vi "testcases.vi"() -> ()   [LabVIEW 2025]
uses:
  <vilib>/LabVIEW Interface for Arduino/Type Defs/Pin Mode.ctl
  <vilib>/LabVIEW Interface for Arduino/LabVIEW Interface for Arduino.lvlib
panel:
  in  "stop":bool
  out "error out":errorcluster
  in  "Board":refnum<visa-resource-name>
  in  "Test cases":T1(ring)
  in  "Tab Control":T2(tab)
  in  "pin":u8
  in  "input val":u8
  out "Value":u8
  out "Outputs":bool[](array[boolean])
  in  "Set values":bool[](array[boolean])
  out "Voltage":dbl(knob) scale=0.0..5.0
  in  "Analog Input Pin (0)":u8
  out "Analog Port":dbl[](array[numeric])
  out "Waveform Chart":dbl(graph)
  in  "PWM 0 (0-255)":u8
  in  "PWM 1 (0-255)":u8
  in  "PWM 2 (0-255)":u8
  in  "PWM Pins":u8[](array[numeric])
  in  "Analog Input Pin":u8
  in  "pwm write single":u8
  in  "PWM Pin single":u8=3
  # "Arduino v4 tests"
  # "0x00 and 0x01 definitely work since every other case requires init and close to function"
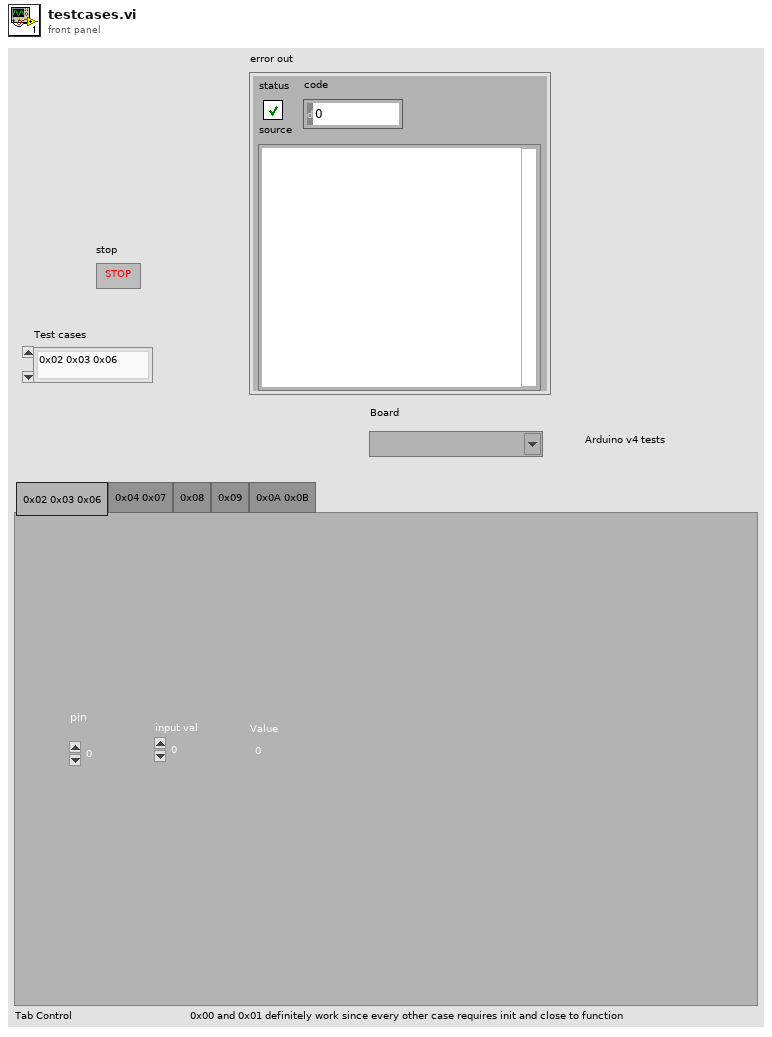
[diagram p1: front panel]
types:
  T1 = enum16{"0x02 0x03 0x06", "0x04 0x07", "0x08", "0x09", "0x0A 0x0B"}
  T2 = enum32{"0x02 0x03 0x06", "0x04 0x07", "0x08", "0x09", "0x0A 0x0B"}
  T3 = typedef "LabVIEW Interface for Arduino.lvlib/Arduino Resource.ctl" = cluster{"VISA resource":refnum<visa-resource-name>, "Board Type":T4, "Connection Type":enum8{"USB / Serial"}, "Bytes Per Packet (15)":u8}
  T4 = typedef "LabVIEW Interface for Arduino.lvlib/Board Type.ctl" = enum16{"Uno", "Dimuelanove w/Atmega 328", "Mega 2560"}
  T5 = typedef "LabVIEW Interface for Arduino.lvlib/Pin Mode.ctl" = enum8{"Input", "Output"}
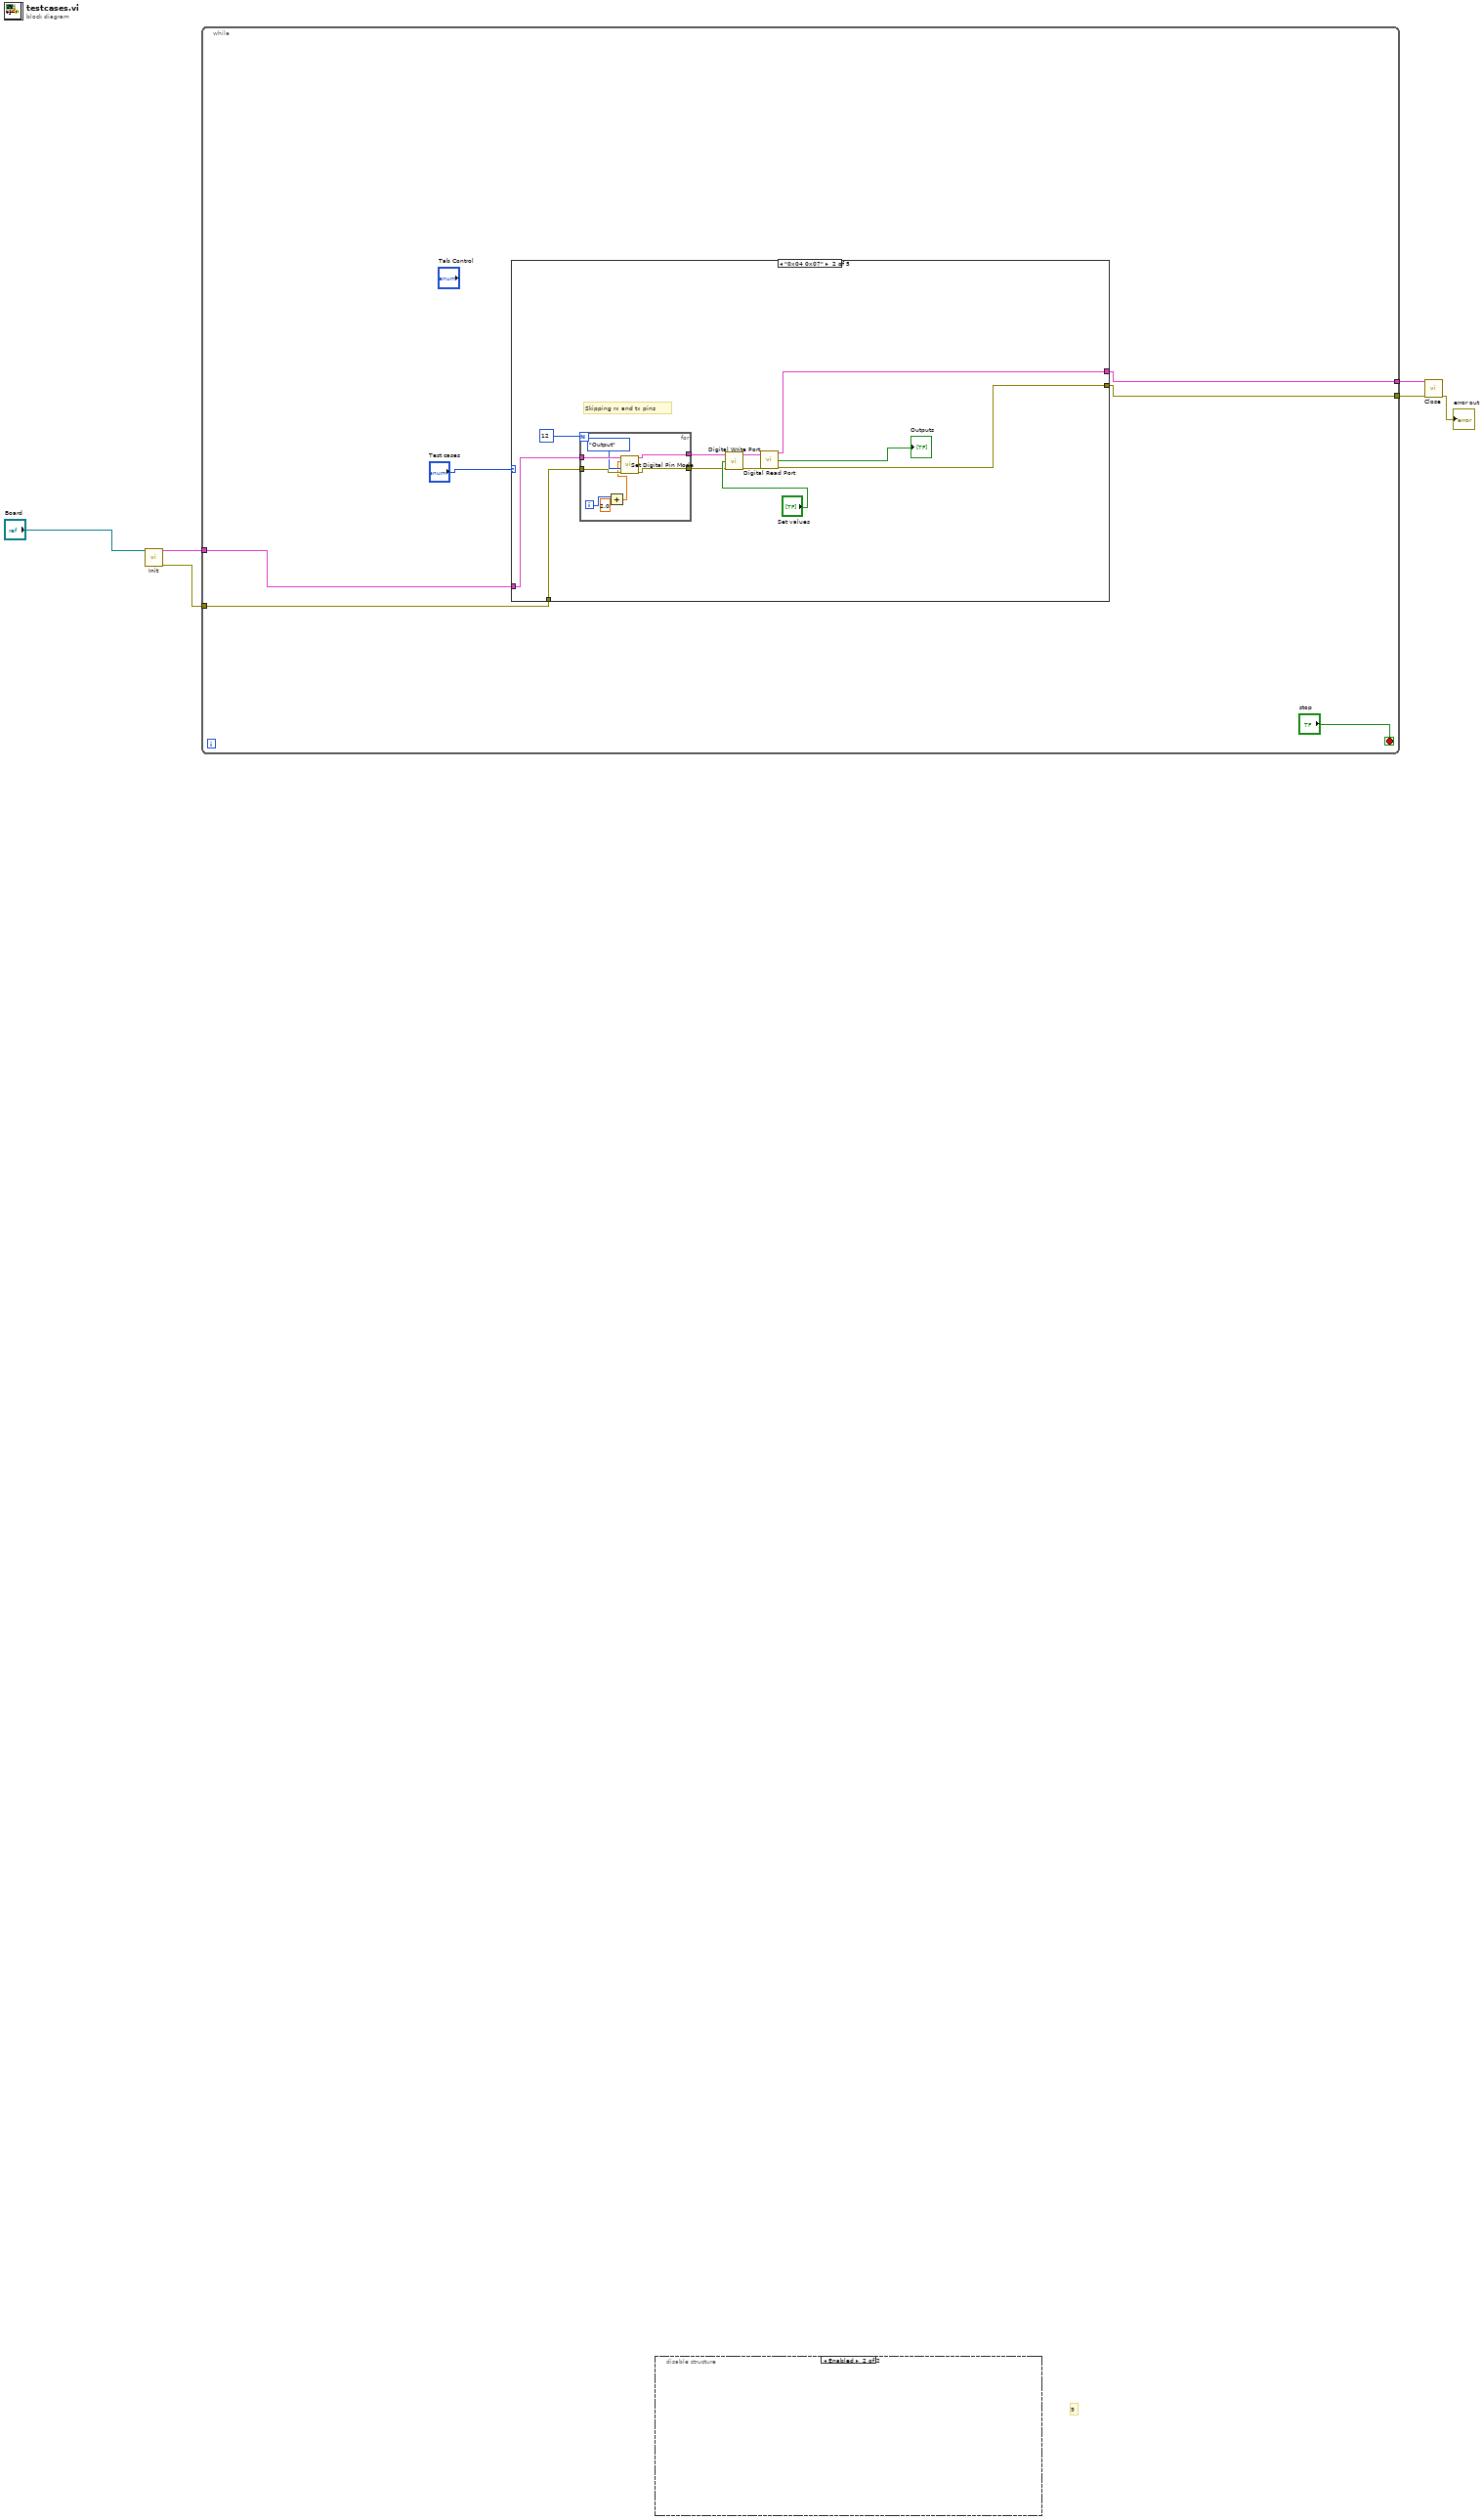
[diagram p0: block diagram]
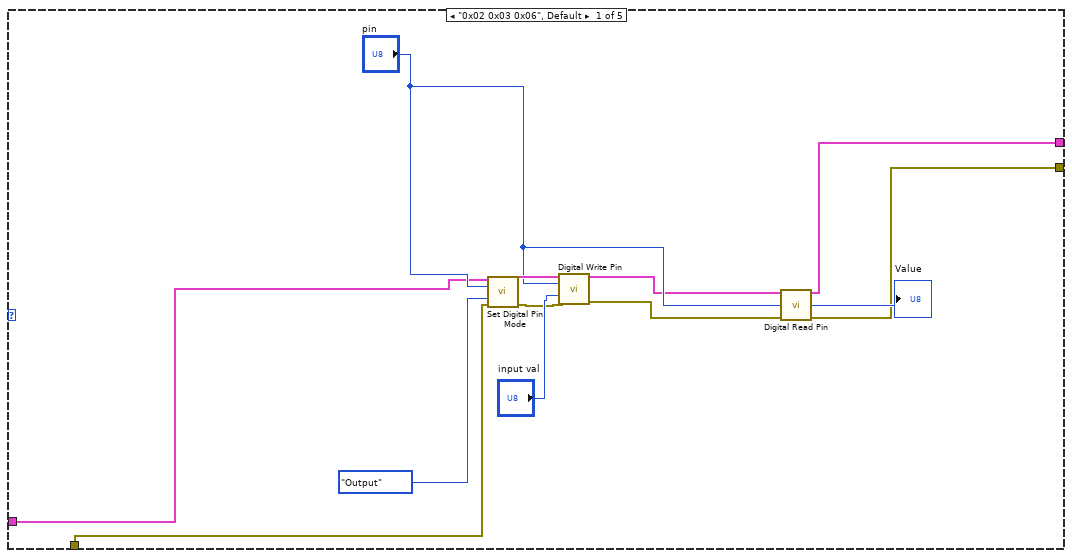
[diagram p2: hidden frame]
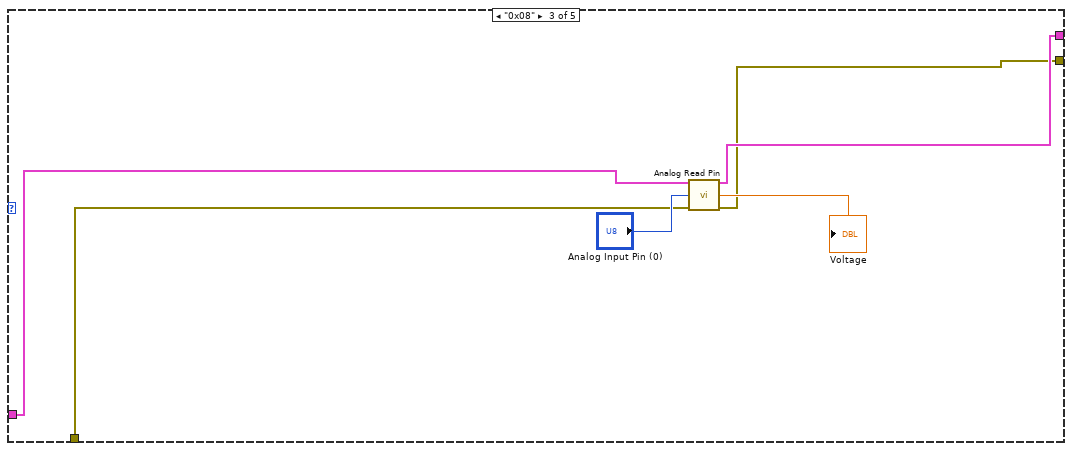
[diagram p3: hidden frame]
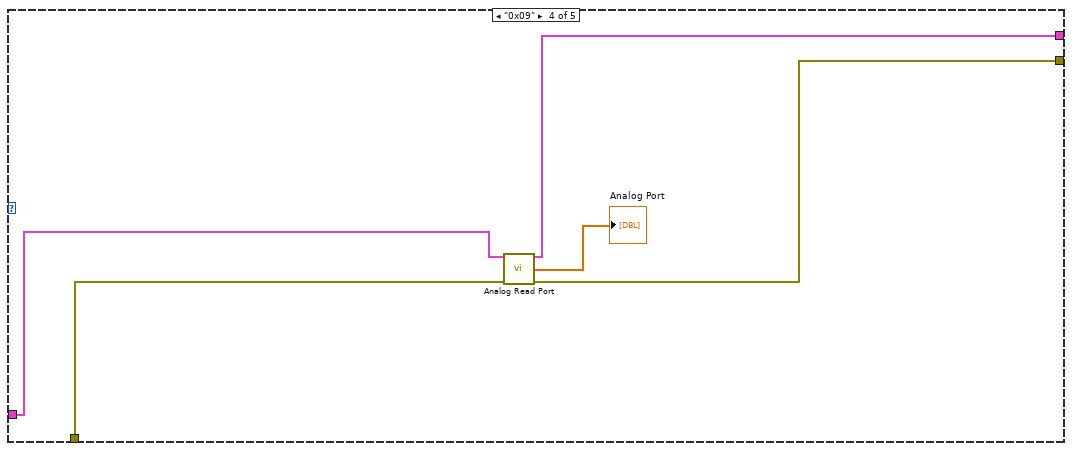
[diagram p4: hidden frame]
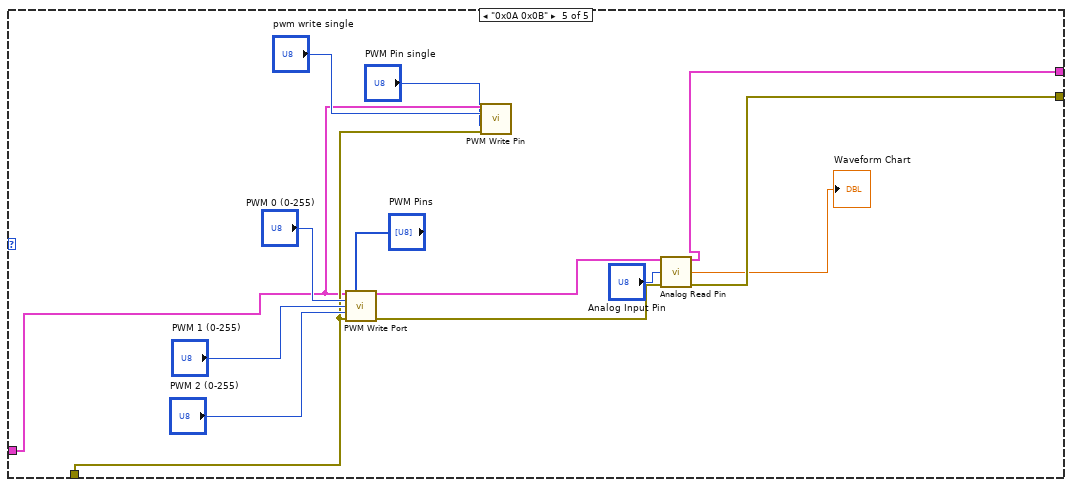
[diagram p5: hidden frame]
diagram:
  # "9"
  n1 = call <vilib>:"Init.vi"("VISA resource"="Board") -> ("Arduino Resource"=w2:T3, "error out"=w1:errorcluster)  [unwired: 17 in]
  n2 = while {
    tunnel: [w10] -> w5
    tunnel: [w9] -> w4
    tunnel: w2 -> [w8]
    tunnel: w1 -> [w7]
    stop <- "stop" stop-if-true
    n3 = case shown="\"0x04 0x07\"" "Test cases" {
      tunnel: w8 -> [w17 w28 w47 w52 w56]
      tunnel: [w16 w35 w46 w53 w61] -> w10
      tunnel: [w15 w32 w45 w50 w62] -> w9
      tunnel: w7 -> [w14 w29 w44 w51 w57]
      frame "0x02 0x03 0x06", Default {
        n4 = call <vilib>:"Set Digital Pin Mode.vi"("Arduino Resource"=w17, "Digital I/O Pin"="pin", "Pin Mode (Input)"=Pin_Mode."Output", "error in"=w14) -> ("Arduino Resource"=w22:T3, "error out"=w13:errorcluster)  [unwired: 10 in]
        n5 = call <vilib>:"Digital Write Pin.vi"("Arduino Resource"=w22, "Digital I/O Pin (0)"="pin", "Value (0)"="input val", "error in"=w13) -> ("Arduino Resource"=w19:T3, "error out"=w18:errorcluster)  [unwired: 10 in]
        n6 = call <vilib>:"Digital Read Pin.vi"("Arduino Resource"=w19, "Digital I/O Pin (0)"="pin", "error in"=w18) -> ("Arduino Resource"=w16:T3, "Value"=→"Value":u8, "error out"=w15:errorcluster)  [unwired: 10 in]
      }
      frame "0x04 0x07" {
        # "Skipping rx and tx pins"
        n7 = for {
          N: 12 -> [_]
          tunnel: w29 -> [w43]
          tunnel: w28 -> [w42]
          tunnel: [w40] -> w27
          tunnel: [w39] -> w26
          i -> [w37]
          n8 = Add(x=w37, y=2.0) -> (x+y=w36:dbl)
          n9 = call <vilib>:"Set Digital Pin Mode.vi"("Arduino Resource"=w42, "Digital I/O Pin"=w36, "Pin Mode (Input)"=Pin_Mode."Output", "error in"=w43) -> ("Arduino Resource"=w40:T3, "error out"=w39:errorcluster)  [unwired: 10 in]
        }
        n10 = call <vilib>:"Digital Write Port.vi"("Arduino Resource"=w27, "Pin Values"="Set values", "error in"=w26) -> ("Arduino Resource"=w31:T3, "error out"=w30:errorcluster)  [unwired: 11 in]
        n11 = call <vilib>:"Digital Read Port.vi"("Arduino Resource"=w31, "error in"=w30) -> ("Arduino Resource"=w35:T3, "Digital Port"=→"Outputs":bool[], "error out"=w32:errorcluster)  [unwired: 11 in]
      }
      frame "0x08" {
        n12 = call <vilib>:"Analog Read Pin.vi"("Arduino Resource"=w47, "Analog Input Pin (0)"="Analog Input Pin (0)", "error in"=w44) -> ("Arduino Resource"=w46:T3, "Voltage"=→"Voltage":dbl, "error out"=w45:errorcluster)  [unwired: 10 in]
      }
      frame "0x09" {
        n13 = call <vilib>:"Analog Read Port.vi"("Arduino Resource"=w52, "error in"=w51) -> ("Arduino Resource"=w53:T3, "Analog Port"=→"Analog Port":dbl[], "error out"=w50:errorcluster)  [unwired: 11 in]
      }
      frame "0x0A 0x0B" {
        n14 = call <vilib>:"PWM Write Port.vi"("Arduino Resource"=w56, "PWM Pins"="PWM Pins", "PWM 0 (0-255)"="PWM 0 (0-255)", "PWM 1 (0-255)"="PWM 1 (0-255)", "PWM 2 (0-255)"="PWM 2 (0-255)", "error in"=w57) -> ("Arduino Resource"=w64:T3, "error out"=w63:errorcluster)  [unwired: 7 in, 1 out]
        n15 = call <vilib>:"PWM Write Pin.vi"("Arduino Resource"=w56, "Duty Cycle (0 - 255)"="pwm write single", "PWM Pin (3)"="PWM Pin single", "error in"=w57) -> ()  [unwired: 10 in, 2 out]
        n16 = call <vilib>:"Analog Read Pin.vi"("Arduino Resource"=w64, "Analog Input Pin (0)"="Analog Input Pin", "error in"=w63) -> ("Arduino Resource"=w61:T3, "Voltage"=→"Waveform Chart":dbl, "error out"=w62:errorcluster)  [unwired: 10 in]
      }
    }
  }
  n17 = disable-structure shown="Enabled" {
    frame Disabled {
    }
    frame Enabled {
    }
  }
  n18 = call <vilib>:"Close.vi"("Arduino Resource"=w5, "error in"=w4) -> ("error out"=→"error out":errorcluster)  [unwired: 13 in]
